vi "MCSA Spectra (N Motors).vi"(0 "waveforms":waveform(dbl)[](array[waveform]), 2 "reset? (F)":bool, 7 "spectrum settings":T3={"number of lines"=15000, "% overlap"=0.0, "maximum frequency [Hz]"=250.0}, 11 "error in (no error)":errorcluster, 12 "demodulation settings":cluster{"enable? (F)":bool, "algorithm":T1}={"enable? (F)"=FALSE, "algorithm"=enum."3-phase signals"}) -> (3 "new spectra available?":bool, 4 "spectrum information":T2, 15 "error out":errorcluster)   [LabVIEW 2014, in "NI_EP_Motor Monitoring.lvlib"]
doc: "Calculates the zoom fast Fourier Transform (FFT) spectra of the motor. You must manually select the polymorphic instance you want to use."
uses:
  <vilib>/addons/Electrical Power/Motor Monitoring/NI_EP_Motor Monitoring.lvlib
  <vilib>/addons/Electrical Power/Motor Monitoring/subVIs/ep_Spectra Settings.ctl
  <vilib>/addons/Electrical Power/Motor Monitoring/subVIs/ep_Demodulation Algorithm.ctl
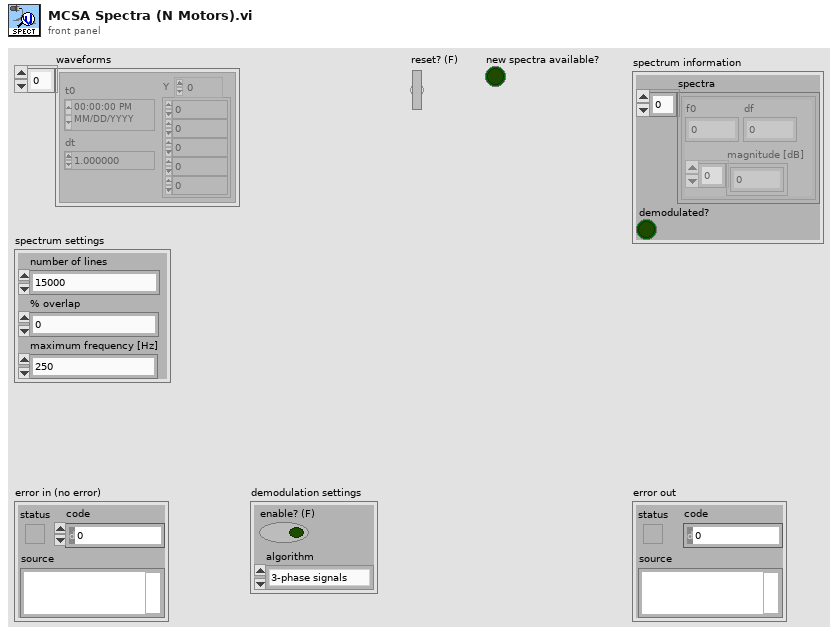
[diagram p1: front panel]
types:
  T1 = typedef "NI_EP_Motor Monitoring.lvlib/ep_Demodulation Algorithm.ctl" = enum16{"1-phase signal", "3-phase signals"}
  T2 = cluster{"spectra":cluster{"f0":dbl, "df":dbl, "magnitude [dB]":dbl[]}[], "demodulated?":bool}
  T3 = typedef "NI_EP_Motor Monitoring.lvlib/ep_Spectra Settings.ctl" = cluster{"number of lines":i32, "% overlap":dbl, "maximum frequency [Hz]":dbl}
  T4 = cluster{"demodulation settings":cluster{"enable? (F)":bool, "algorithm":T1}, "dt":dbl, "block size":i32}
  T5 = typedef "NI_EP_Motor Monitoring.lvlib/ep_Initial Conditions for MCSA Spectra.ctl" = cluster{"hilbert state":cluster{"delay conditions":dbl[], "filter conditions":dbl[]}, "zoom FFT state":cluster{"phase state":dbl, "zoom FFT state":cluster{"zoom settings state":cluster{"zoom":i32, "stop band attenuation":enum16{"84 dB", "96 dB", "120 dB"}, "alias protect in final transition":bool, "oversampling ratio":dbl}, "SML Decimation Filter (complex input) state":cluster{"decimation settings state":cluster{"M":i32, "stop band attenuation":enum16{"84 dB", "96 dB", "120 dB"}, "alias protect in transition band":bool, "oversampling ratio":dbl}, "counter for garbage samples state":i32, "sml_Parameter Setting for Zoom Factor state":cluster{"filter length * interpolation state":i32, "interpolation state":i32, "comb filter order state":i32, "CFIR par state":cluster{"h":dbl[], "M":i32, "N":i32}, "LFIR par state":cluster{"h":dbl[], "M":i32, "N":i32}, "CIC Stages state":i32}, "aal_CIC (complex input) state":cluster{"aal_cascaded moving average (complex input) state":cluster{"states":cdb[], "circular buffers state":cdb[][], "circular buffer counter state":i32}, "aal_moving average with decimation by order (complex input) state":cluster{"residue result state":cdb, "processed data counter state":i32}}, "sml_Cascaded Decimation Filter (complex input) CFIR state":cluster{"unprocessed data state":cdb[], "final conditions state":cdb[][], "sml_M-1 Decimator with IC (complex input) state":cluster{"coefficients in reverse order state":dbl[], "max index for coefficients state":i32}}, "sml_Cascaded Decimation Filter (complex input) LFIR state":cluster{"unprocessed data state":cdb[], "final conditions state":cdb[][], "sml_M-1 Decimator with IC (complex input) state":cluster{"coefficients in reverse order state":dbl[], "max index for coefficients state":i32}}}, "ma_SML Data Packing (complex input) state":cluster{"array getting packed state":cdb[], "last array processed state":cdb[], "index state":i32, "packing parameters state":cluster{i32, "size":i32}}}, "FFT{X} [Vrms]":cdb[]}, "IIR filter state":cluster{"filter state":dbl[]}, "demodulation settings":cluster{"enable? (F)":bool, "algorithm":T1}, "highpass IIR Filter":cluster{"filter structure":enum32{"IIR 2nd Order", "IIR 4th Order"}, "Reverse Coefficients":dbl[], "Forward Coefficients":dbl[]}, "Hilbert FIR filter":cluster{"coefficients":dbl[], "delay":i32}, "zoom FFT settings":T6}
  T6 = typedef "NI_EP_Motor Monitoring.lvlib/ep_Zoom FFT Settings.ctl" = cluster{"FFT settings":cluster{"window":u16, "Window Size":i32, "FFT Size":i32, "%overlap":dbl}, "zoom settings":cluster{"zoom":i32, "stop band attenuation":enum16{"84 dB", "96 dB", "120 dB"}, "alias protect in final transition":bool, "oversampling ratio":dbl}, "other settings":cluster{"fmod":dbl, "f0":dbl, "df":dbl, "oidx":i32, "olen":i32}, "iterations":i32, "max block size":i32, "fs":dbl}
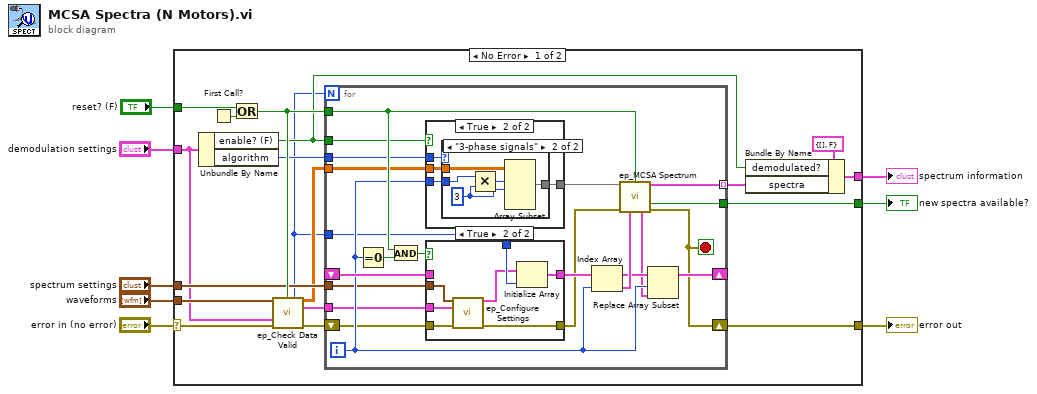
[diagram p0: block diagram]
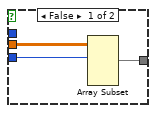
[diagram p2: hidden frame]
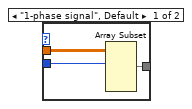
[diagram p3: hidden frame]
diagram:
  n1 = case shown="No Error" "error in (no error)" {
    selector: "error in (no error)" -> [w20 w72]
    tunnel: [w23 w72] -> w5
    tunnel: "waveforms" -> [w17 _]
    tunnel: "reset? (F)" -> [w26 _]
    tunnel: "spectrum settings" -> [w13 _]
    tunnel: "demodulation settings" -> [w9 _]
    tunnel: [w24 _] -> w2
    tunnel: [w21 _] -> w1
    frame No Error {
      n2 = Unbundle By Name(w9) -> ("enable? (F)"=w15:bool, "algorithm"=w16:T1)
      n3 = First Call?() -> (First Call?: T/F=w25:bool)
      n4 = Or(x=w26, y=w25) -> (x .or. y?=w19:bool)
      n5 = call <vilib>:"ep_Check Data Valid.vi"("waveforms"=w17, "reset? (F)"=w19, "demodulation settings"=w9, "error in (no error)"=w20) -> ("number of spectra"=w10:i32, "signals"=w11:dbl[][], "parameters"=w12:T4, "error out"=w18:errorcluster)  [unwired: 8 in]
      n6 = for {
        N: w10 -> [_]
        shift-right: [w45] -> _
        shift-left: _ -> [w46]
        shift-right: [w33] -> w23
        shift-left: w18 -> [w32]
        tunnel: w19 -> [w40]
        tunnel: w11 -> [w38]
        tunnel: [w34] -> w24
        tunnel: [w47] -> w14 mode=indexing
        tunnel: w16 -> [w35]
        tunnel: w15 -> [w36]
        tunnel: w13 -> [w31]
        tunnel: w12 -> [w30]
        tunnel: w10 -> [w29]
        i -> [w39]
        stop <- w33 stop-if-true
        n7 = Equal To 0?(x=w39) -> (x = 0?=w42:bool)
        n8 = And(x=w40, y=w42) -> (x .and. y?=w41:bool)
        n9 = case shown="True" w36 {
          tunnel: w39 -> [w48 w53]
          tunnel: w38 -> [w50 w54]
          tunnel: [w49 w52] -> w37
          tunnel: w35 -> [_ w51]
          frame False {
            n10 = Array Subset(array=w50, index (row)=w48) -> (w49:dbl[][])  [unwired: 3 in]
          }
          frame True {
            n11 = case shown="\"3-phase signals\"" w51 {
              tunnel: w54 -> [w57 w62]
              tunnel: w53 -> [w56 w61]
              tunnel: [w55 w58] -> w52
              frame "1-phase signal", Default {
                n12 = Array Subset(array=w57, index (row)=w56) -> (w55:dbl[][])  [unwired: 3 in]
              }
              frame "3-phase signals" {
                w59 = 3 ("y")
                n13 = Multiply(x=w61, y=w59) -> (x*y=w60:i32)
                n14 = Array Subset(array=w62, index (row)=w60, length (row)=w59) -> (w58:dbl[][])  [unwired: 2 in]
              }
            }
          }
        }
        n15 = case shown="True" w41 {
          tunnel: w46 -> [w64 _]
          tunnel: [w64 w67] -> w43
          tunnel: w29 -> [_ w71]
          tunnel: w32 -> [w63 w70]
          tunnel: w31 -> [_ w69]
          tunnel: w30 -> [_ w68]
          tunnel: [w63 w66] -> w28
          frame False {
          }
          frame True {
            n16 = call <vilib>:"ep_Configure Settings.vi"("spectra settings"=w69, "parameters"=w68, "error in (no error)"=w70) -> ("initial conditions"=w65:T5, "error out"=w66:errorcluster)  [unwired: 11 in]
            n17 = Initialize Array(w65, w71) -> (w67:T5[])
          }
        }
        n18 = Index Array(array=w43, index=w39) -> (element=w44:T5)
        n19 = call <vilib>:"ep_MCSA Spectrum.vi"("signals"=w37, "reset? (F)"=w40, "error in (no error)"=w28, "initial conditions"=w44) -> ("FFT magnitude"=w47:cluster{"f0":dbl, "df":dbl, "spectrum":dbl[]}, "spectrum ready?"=w34:bool, "final conditions"=w27:T5, "error out"=w33:errorcluster)  [unwired: 7 in, 1 out]
        n20 = Replace Array Subset(array=w43, new element=w27, index=w39) -> (w45:T5[])
      }
      n21 = Bundle By Name(cluster=T2 {"spectra"=[], "demodulated?"=FALSE} ("spectra information"), "demodulated?"=w15, "spectra"=w14) -> (w21:T2)
    }
    frame Error {
    }
  }
  "spectrum information" <- w1
  "new spectra available?" <- w2
  "error out" <- w5
